vi "CUIT553.vi"(4 "Error In":errorcluster, 7 "Command":string) -> (0 "Error Out":errorcluster, 3 "Response":string)   [LabVIEW 2018]
uses:
  MOKO_LabViewLibrary/MokoLowLevel/MokoLowLovelControl/MLLC_ConnectCluster.ctl
  MOKO_LabViewLibrary/MokoLowLevel/MokoLowLovelControl/MLLC_InterfaceType.ctl
  MOKO_LabViewLibrary/MokoLowLevel/MokoLowLovelControl/MLLC_OpenedSession.ctl
  MOKO_LabViewLibrary/MokoLowLevel/MokoLowLovelControl/MLLC_InterfaceSettings.ctl
  MOKO_LabViewLibrary/MokoLowLevel/MokoLowLovelControl/MLLC_InterfaceKind.ctl
  data/CUIT553_COMMANDs_driver.ctl
panel:
  in  "Settings":T6={"Saved Data"=variant, "Permanent data"={"Connect"={"InterfaceType"=enum."VISA", "OpenedSession"="", "InterfaceSettings"={"Interface"=enum."RS232", "EOS 4 read"=enum."LF (\\n)", "EOS 4 write"=enum."LF (\\n)", "TMO, ms"=10000, "Sett"=variant(cluster{"Baud Rate":u32, "Data Bits":u16, "Parity":u16, "Stop Bits":u16, "Flow Control":u16, "Eho":bool} {"Baud Rate"=75, "Data Bits"=0, "Parity"=0, "Stop Bits"=0, "Flow Control"=0, "Eho"=FALSE})}}, "Value"={"I"=0.0, "P"=0.0, "T"=0.0}, "String"="empty"}}
  in  "Error Code":u32
  in  "Driver Name":string="CUIT553"
  in  "Mode":T7(ring)=enum."Check"
  # "CUIT553"
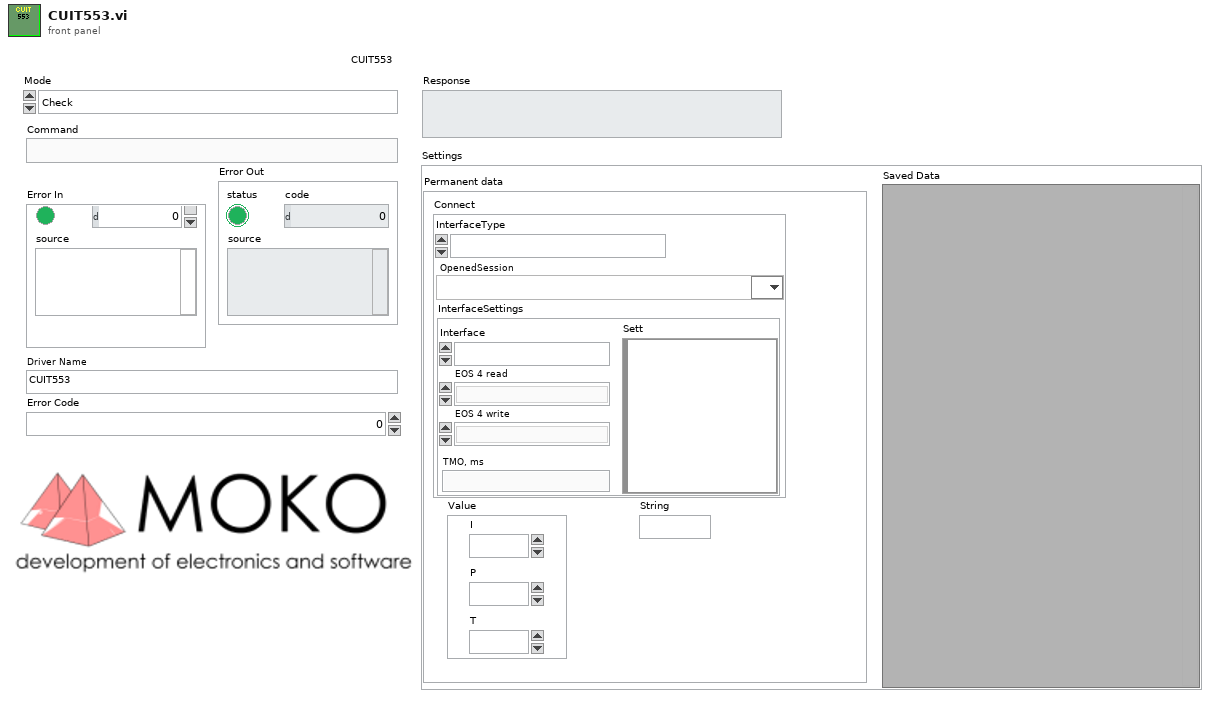
[diagram p1: front panel]
types:
  T1 = typedef "MLLC_ConnectCluster.ctl" = cluster{"InterfaceType":T2, "OpenedSession":T3, "InterfaceSettings":T4}
  T2 = typedef "MLLC_InterfaceType.ctl" = enum16{"VISA", "Prologix USB-GPIB"}
  T3 = typedef "MLLC_OpenedSession.ctl" = refnum<visa-resource-name>
  T4 = typedef "MLLC_InterfaceSettings.ctl" = cluster{"Interface":T5, "EOS 4 read":enum16{"Default (=EOS 4 write)", "CR (\\r)", "LF (\\n)", "None"}, "EOS 4 write":enum16{"CR+LF (\\r\\n)", "CR (\\r)", "LF (\\n)", "None"}, "TMO, ms":i32, "Sett":variant}
  T5 = typedef "MLLC_InterfaceKind.ctl" = enum16{"RS232", "GPIB", "USB", "Ethernet", "another"}
  T6 = cluster{"Saved Data":variant, "Permanent data":cluster{"Connect":T1, "Value":cluster{"I":dbl, "P":dbl, "T":dbl}, "String":string}}
  T7 = enum16{"get", "set", "close", "Init", "Check", "ID"}
  T8 = cluster{"Connect":T1, "Value":cluster{"I":dbl, "P":dbl, "T":dbl}, "String":string}
  T9 = typedef "MLLC_Mode.ctl" = enum16{"get", "set", "close", "Init", "Check"}
  T10 = typedef "CUIT553_COMMANDs_driver.ctl" = enum16{"empty", "INIT", "T1T2", "T2T3", "T3T4", "T4T5", "T5P1", "P1P2", "P2P3", "P3", "ROUNDS", "RPM", "RESET", "DRAIN READ", "DRAIN CONTROL"}
  T11 = typedef "MLLC_Error.ctl" = errorcluster
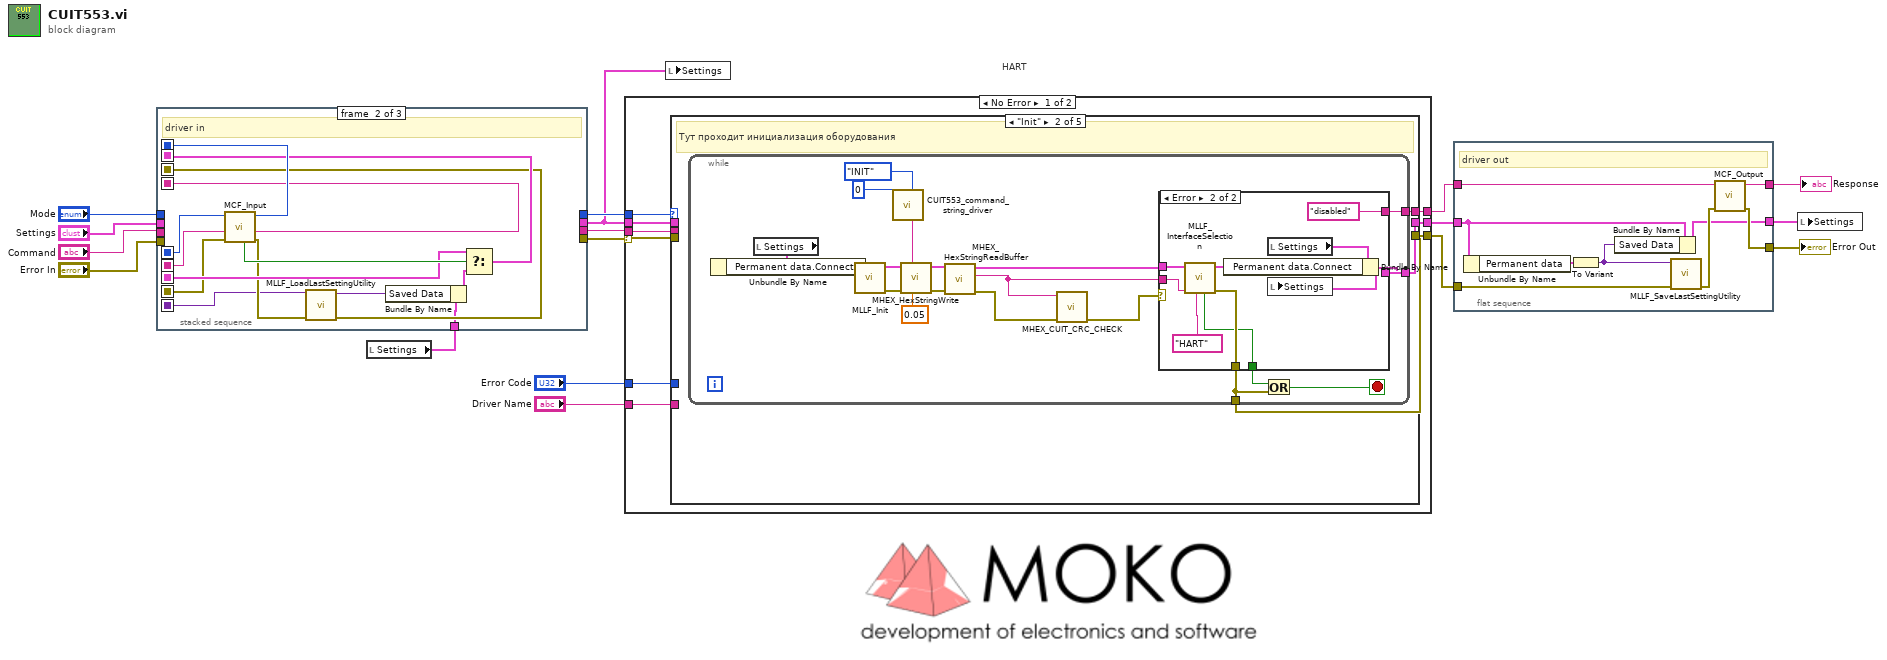
[diagram p0: block diagram]
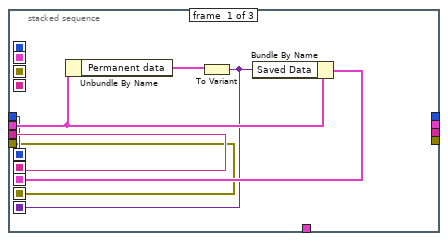
[diagram p2: hidden frame]
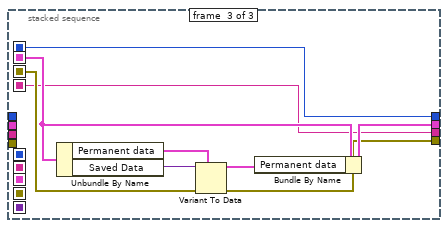
[diagram p3: hidden frame]
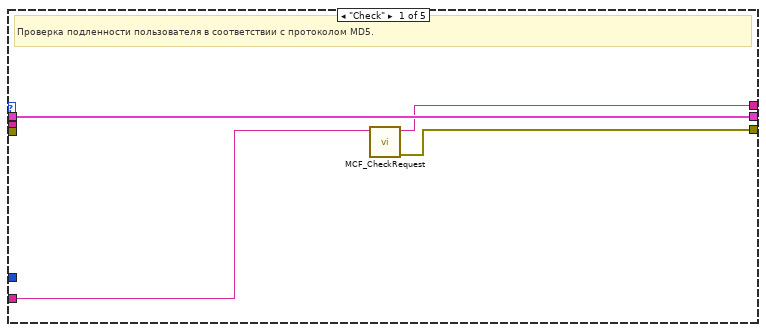
[diagram p4: hidden frame]
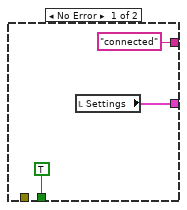
[diagram p5: hidden frame]
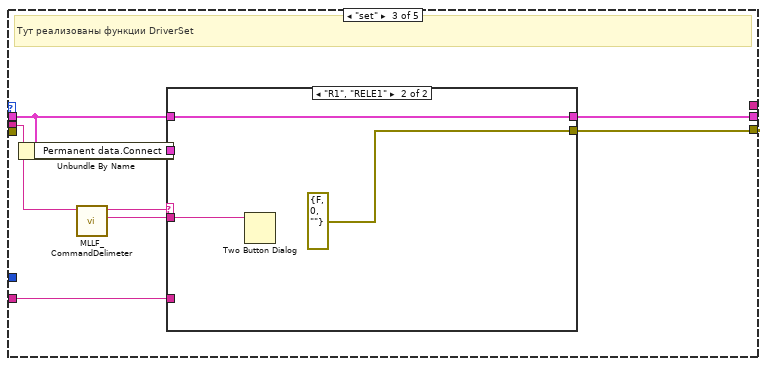
[diagram p6: hidden frame]
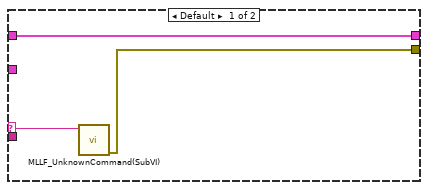
[diagram p7: hidden frame]
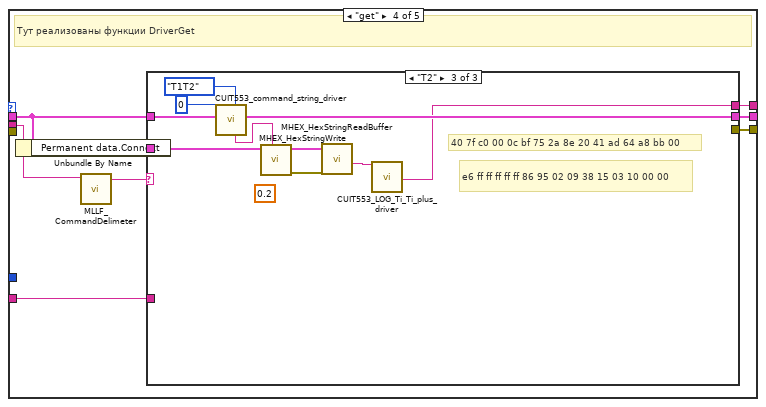
[diagram p8: hidden frame]
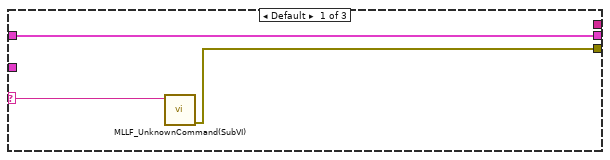
[diagram p9: hidden frame]
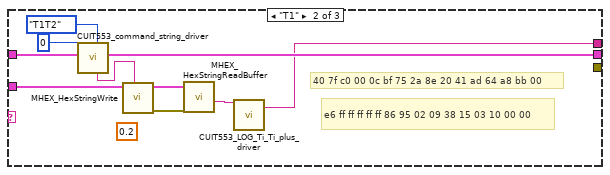
[diagram p10: hidden frame]
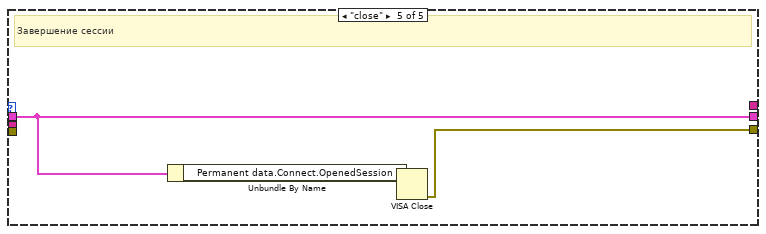
[diagram p11: hidden frame]
diagram:
  # "HART"
  n1 = local read "Settings"() -> (w1:T6)
  n2 = stacked-sequence {
    seq-local: [w20 _ _] -> [_ w36 _]
    seq-local: [w19 _ _] -> [_ w37 _]
    seq-local: [w22 _ _] -> [_ w32 _]
    seq-local: [w18 _ _] -> [_ w31 _]
    seq-local: [w21 _ _] -> [_ w27 _]
    seq-local: [_ w28 _] -> [_ _ w44]
    seq-local: [_ w38 _] -> [_ _ w41]
    seq-local: [_ w35 _] -> [_ _ w40]
    seq-local: [_ w34 _] -> [_ _ w45]
    tunnel: "Command" -> [w20 _ _]
    tunnel: "Mode" -> [w19 _ _]
    tunnel: "Error In" -> [w18 _ _]
    tunnel: "Settings" -> [w23 _ _]
    tunnel: w1 -> [_ w26 _]
    tunnel: [_ _ w40] -> w3
    tunnel: [_ _ w43] -> w4
    tunnel: [_ _ w42] -> w2
    tunnel: [_ _ w41] -> w5
    frame #0 {
      n3 = Unbundle By Name(w23) -> ("Permanent data"=w24:T8)
      n4 = To Variant(anything=w24) -> (Variant=w21:variant)
      n5 = Bundle By Name(cluster=w23, "Saved Data"=w21) -> (w22:T6)
    }
    frame #1 {
      # "driver in"
      n6 = call "MCF_Input.vi"("Error In"=w31, "Command in"=w36, "Mode in"=w37) -> ("Error Out"=w30:errorcluster, "Command out"=w35:string, "Mode out"=w38:T9, "Boolean"=w33:bool)  [unwired: 5 in]
      n7 = call "MLLF_LoadLastSettingUtility.vi"("Error In"=w30, "Save data in"=w27) -> ("Error Out"=w28:errorcluster, "Save data out"=w25:variant)  [unwired: 8 in]
      n8 = Bundle By Name(cluster=w26, "Saved Data"=w25) -> (w29:T6)
      n9 = Select(t=w32, s=w33, f=w29) -> (s? t:f=w34:T6)
    }
    frame #2 {
      n10 = Unbundle By Name(w45) -> ("Permanent data"=w46:T8, "Saved Data"=w39:variant)
      n11 = Variant To Data(error in=w44, type=w46, Variant=w39) -> (data=w47:T8, error out=w42:errorcluster)
      n12 = Bundle By Name(cluster=w45, "Permanent data"=w47) -> (w43:T6)
    }
  }
  n13 = case shown="No Error" w2 {
    selector: w2 -> [w53 w142]
    tunnel: [w48 w142] -> w9
    tunnel: w5 -> [w56 _]
    tunnel: [w55 _] -> w11
    tunnel: w3 -> [w54 _]
    tunnel: w4 -> [w50 w141]
    tunnel: "Error Code" -> [w52 _]
    tunnel: "Driver Name" -> [w51 _]
    tunnel: [w49 w141] -> w10
    frame No Error {
      n14 = case shown="\"Init\"" w56 {
        tunnel: [w58 w62 _ w110 _] -> w55
        tunnel: w54 -> [_ _ w98 w113 _]
        tunnel: w53 -> [_ _ _ _ _]
        tunnel: w52 -> [_ _ _ _ _]
        tunnel: w51 -> [w59 _ w100 w111 _]
        tunnel: w50 -> [w60 _ w102 w116 w139]
        tunnel: [w60 w63 w101 w115 w139] -> w49
        tunnel: [w57 w61 w95 w109 w138] -> w48
        frame "Check" {
          # "Проверка подленности пользователя в соответствии с протоколом MD5."
          n15 = call "MCF_CheckRequest.vi"("Driver Name"=w59) -> ("Error Out"=w57:errorcluster, "Output String"=w58:string)  [unwired: 9 in]
        }
        frame "Init" {
          # "Тут проходит инициализация оборудования"
          n16 = while {
            tunnel: [w79] -> w63
            tunnel: [w77] -> w62
            tunnel: [w70] -> w61
            stop <- w81 stop-if-true
            n17 = local read "Settings"() -> (w80:T6)
            n18 = Unbundle By Name(w80) -> ("Permanent data.Connect"=w78:T1)
            n19 = call "MLLF_Init.vi"("DriverConnect in"=w78) -> ("Error Out"=w74:errorcluster, "DriverConnect out"=w75:T1)  [unwired: 7 in]
            n20 = call "CUIT553_command_string_driver.vi"("command"=CUIT553_COMMANDs_driver."INIT", "adress"=0) -> ("comand out"=w67:string)  [unwired: 7 in, 2 out]
            n21 = call "MHEX_HexStringWrite.vi"("Delay Time (s)"=0.05, "Command"=w67, "error in"=w74, "DriverConnect in"=w75) -> ("error out"=w72:T11, "DriverConnect out"=w73:T1)  [unwired: 6 in]
            n22 = call "MHEX_HexStringReadBuffer.vi"("error in"=w72, "DriverConnect in"=w73) -> ("error out"=w65:T11, "String from device out"=w64:string, "DriverConnect out"=w71:T1)  [unwired: 6 in, 1 out]
            n23 = call "MHEX_CUIT_CRC_CHECK.vi"("Error In"=w65, "string in"=w64) -> ("Error Out"=w66:errorcluster)  [unwired: 9 in]
            n24 = case shown="Error" w66 {
              tunnel: w71 -> [_ w93]
              tunnel: [TRUE w88] -> w82
              tunnel: [_ w94] -> w70
              tunnel: [w84 w89] -> w79
              tunnel: ["connected" "disabled"] -> w77
              tunnel: w64 -> [_ w86]
              frame No Error {
                n25 = local read "Settings"() -> (w84:T6)
              }
              frame Error {
                n26 = call "MLLF_InterfaceSelection.vi"("Driver Name"="HART" ("String"), "Answer:"=w86, "DriverConnect in"=w93) -> ("error out"=w94:T11, "DriverConnect out"=w91:T1, "stop init?"=w88:bool)  [unwired: 4 in, 2 out]
                n27 = local read "Settings"() -> (w90:T6)
                n28 = Bundle By Name(cluster=w90, "Permanent data.Connect"=w91) -> (w89:T6)
                n29 = local write "Settings"(w89) -> ()
              }
            }
            n30 = Or(x=w82, y=w70) -> (x .or. y?=w81:bool)
          }
        }
        frame "set" {
          # "Тут реализованы функции DriverSet"
          n31 = Unbundle By Name(w102) -> ("Permanent data.Connect"=w99:T1)
          n32 = call "MLLF_CommandDelimeter.vi"("command with param"=w98) -> ("param 1"=w96:string, "command"=w97:string)  [unwired: 6 in, 3 out]
          n33 = case shown="\"R1\", \"RELE1\"" w97 {
            selector: w97 -> [w104 _]
            tunnel: [w105 w108] -> w101
            tunnel: w102 -> [w105 w108]
            tunnel: w99 -> [_ _]
            tunnel: w96 -> [_ w106]
            tunnel: [w103 errorcluster {"status"=FALSE, "code"=0, "source"=""} ("error IO")] -> w95
            tunnel: w100 -> [_ _]
            frame Default {
              n34 = call "MLLF_UnknownCommand(SubVI).vi"("Unknown command"=w104) -> ("error out"=w103:errorcluster)  [unwired: 10 in]
            }
            frame "R1", "RELE1" {
              n35 = Two Button Dialog(message=w106) -> ()  [unwired: 2 in, 1 out]
            }
          }
        }
        frame "get" {
          # "Тут реализованы функции DriverGet"
          n36 = Unbundle By Name(w116) -> ("Permanent data.Connect"=w114:T1)
          n37 = call "MLLF_CommandDelimeter.vi"("command with param"=w113) -> ("command"=w112:string)  [unwired: 6 in, 4 out]
          n38 = case shown="\"T2\"" w112 {
            selector: w112 -> [w118 _ _]
            tunnel: w114 -> [_ w125 w134]
            tunnel: w116 -> [w119 w126 w135]
            tunnel: [w119 w126 w135] -> w115
            tunnel: [_ w121 w129] -> w110
            tunnel: [w117 _ _] -> w109
            tunnel: w111 -> [_ _ _]
            frame Default {
              n39 = call "MLLF_UnknownCommand(SubVI).vi"("Unknown command"=w118) -> ("error out"=w117:errorcluster)  [unwired: 10 in]
            }
            frame "T1" {
              (unwired) 0.2 ("Delay Time (s)")
              # "40 7f c0 00 0c bf 75 2a 8e 20 41 ad 64 a8 bb 00"
              # "e6 ff ff ff ff ff 86 95 02 09 38 15 03 10 00 00"
              n40 = call "CUIT553_command_string_driver.vi"("command"=CUIT553_COMMANDs_driver."T1T2", "adress"=0) -> ("comand out"=w122:string)  [unwired: 7 in, 2 out]
              n41 = call "MHEX_HexStringWrite.vi"("Command"=w122, "DriverConnect in"=w125) -> ("error out"=w123:T11, "DriverConnect out"=w124:T1)  [unwired: 8 in]
              n42 = call "MHEX_HexStringReadBuffer.vi"("error in"=w123, "DriverConnect in"=w124) -> ("String from device out HEX"=w120:string)  [unwired: 6 in, 3 out]
              n43 = call "CUIT553_LOG_Ti_Ti_plus_driver.vi"("DATA"=w120) -> ("Ti float"=w121:string)  [unwired: 17 in, 1 out]
            }
            frame "T2" {
              (unwired) 0.2 ("Delay Time (s)")
              # "40 7f c0 00 0c bf 75 2a 8e 20 41 ad 64 a8 bb 00"
              # "e6 ff ff ff ff ff 86 95 02 09 38 15 03 10 00 00"
              n44 = call "CUIT553_command_string_driver.vi"("command"=CUIT553_COMMANDs_driver."T1T2", "adress"=0) -> ("comand out"=w131:string)  [unwired: 7 in, 2 out]
              n45 = call "MHEX_HexStringWrite.vi"("Command"=w131, "DriverConnect in"=w134) -> ("error out"=w132:T11, "DriverConnect out"=w133:T1)  [unwired: 8 in]
              n46 = call "MHEX_HexStringReadBuffer.vi"("error in"=w132, "DriverConnect in"=w133) -> ("String from device out HEX"=w130:string)  [unwired: 6 in, 3 out]
              n47 = call "CUIT553_LOG_Ti_Ti_plus_driver.vi"("DATA"=w130) -> ("Ti plus float"=w129:string)  [unwired: 17 in, 1 out]
            }
          }
        }
        frame "close" {
          # "Завершение сессии"
          n48 = Unbundle By Name(w139) -> ("Permanent data.Connect.OpenedSession"=w140:T3)
          n49 = VISA Close(VISA resource name=w140) -> (error out=w138:errorcluster)  [unwired: 1 in]
        }
      }
    }
    frame Error {
    }
  }
  n50 = local write "Settings"(w4) -> ()
  n51 = flat-sequence {
    tunnel: [w151] -> w8
    tunnel: [w150] -> w6
    tunnel: w11 -> [w149]
    tunnel: w9 -> [w148]
    tunnel: w10 -> [w144]
    tunnel: [w146] -> w7
    frame #0 {
      # "driver out"
      n52 = Unbundle By Name(w144) -> ("Permanent data"=w143:T8)
      n53 = To Variant(anything=w143) -> (Variant=w145:variant)
      n54 = Bundle By Name(cluster=w144, "Saved Data"=w145) -> (w146:T6)
      n55 = call "MLLF_SaveLastSettingUtility.vi"("error in"=w148, "Saved Data"=w145) -> ("error out"=w147:T11)  [unwired: 8 in, 1 out]
      n56 = call "MCF_Output.vi"("Error In"=w147, "Input"=w149) -> ("Error Out"=w150:errorcluster, "Output"=w151:string)  [unwired: 8 in]
    }
  }
  n57 = local write "Settings"(w7) -> ()
  "Response" <- w8
  "Error Out" <- w6
